vi "Write Data String.vi"(8 "error in (no error)":errorcluster, 10 "Data":string, 11 "Project Builder in":refnum<class "Project Builder.lvclass">) -> (0 "error out":errorcluster, 3 "Project Builder out":refnum<class "Project Builder.lvclass">)   [LabVIEW 2020, in "ProjectBuilder.lvlib" / "Project Builder.lvclass"]
uses:
  Project Builder.lvclass
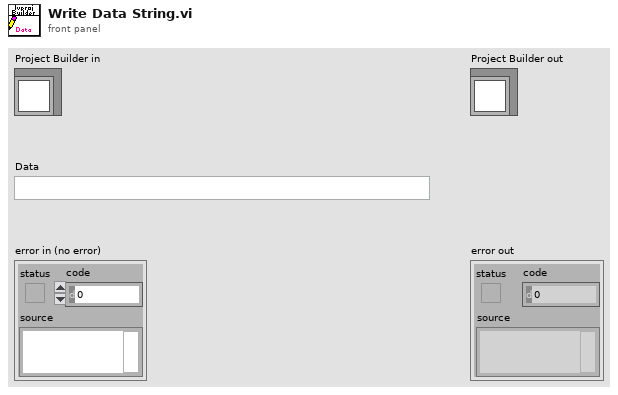
[diagram p1: front panel]
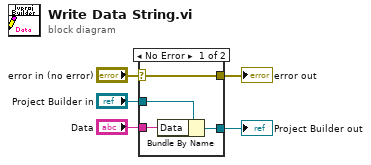
[diagram p0: block diagram]
diagram:
  n1 = case shown="No Error" "error in (no error)" {
    selector: "error in (no error)" -> [w9 w10]
    tunnel: [w9 w10] -> w4
    tunnel: [w7 w11] -> w2
    tunnel: "Project Builder in" -> [w8 w11]
    tunnel: "Data" -> [w6 _]
    frame No Error {
      n2 = Bundle By Name(cluster=w8, "Data"=w6) -> (w7:refnum<class "Project Builder.lvclass">)
    }
    frame Error {
    }
  }
  "error out" <- w4
  "Project Builder out" <- w2
